vi "Read Configuration Change.vi"(8 "error in (no error)":errorcluster, 11 "CIFCorePlugin in":refnum<class "CIFCorePlugin.lvclass">) -> (0 "error out":errorcluster, 2 "Configuration Change":bool, 3 "CIFCorePlugin out":refnum<class "CIFCorePlugin.lvclass">)   [LabVIEW 2021, in "CIFCorePlugin.lvclass"]
uses:
  CIFCorePlugin.lvclass
  CIFCorePlugin.lvclass/CIFCorePlugin.ctl
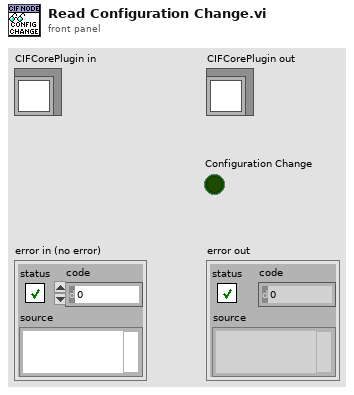
[diagram p1: front panel]
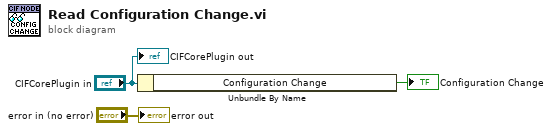
[diagram p0: block diagram]
diagram:
  n1 = Unbundle By Name("CIFCorePlugin in") -> ("Configuration Change"=→"Configuration Change":bool)
  "error out" <- "error in (no error)"
  "CIFCorePlugin out" <- "CIFCorePlugin in"
